vi "Read State DVR.vi"(8 "error in (no error)":errorcluster, 11 "Stabilize Laser in":refnum<class "Stabilize Laser.lvclass">) -> (0 "error out":errorcluster, 2 "State DVR":refnum<data-value>, 3 "Stabilize Laser out":refnum<class "Stabilize Laser.lvclass">)   [LabVIEW 2013, in "Stabilize Laser.lvclass"]
uses:
  Stabilize Laser.lvclass
  Data/cPAS Data.lvclass
  Stabilize Laser.lvclass/Stabilize Laser.ctl
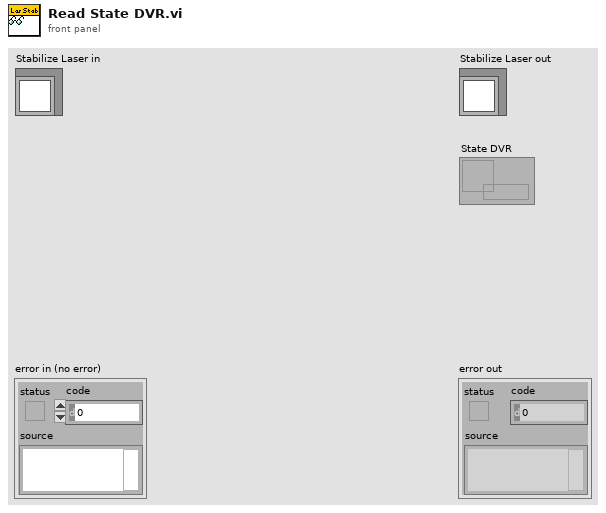
[diagram p1: front panel]
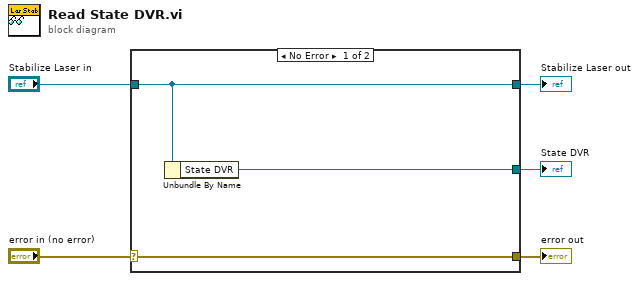
[diagram p0: block diagram]
diagram:
  n1 = case shown="No Error" "error in (no error)" {
    selector: "error in (no error)" -> [w8 w9]
    tunnel: [w8 w9] -> w4
    tunnel: [w7 w10] -> w2
    tunnel: "Stabilize Laser in" -> [w7 w10]
    tunnel: [w6 _] -> w1
    frame No Error {
      n2 = Unbundle By Name(w7) -> ("State DVR"=w6:refnum<data-value>)
    }
    frame Error {
    }
  }
  "error out" <- w4
  "Stabilize Laser out" <- w2
  "State DVR" <- w1
